vi "Tacking Helper Helper - Waypoint Builder.vi"(4 "Second Arm Length":dbl, 5 "Current Waypoint\nBeing Adjusted":i32, 6 "Starting Arm Length":dbl, 7 "Waypoint\nArray In":T1[](array[typedef]), 9 "Second Angle":dbl, 10 "If true, the starting angle was\nthe last angle used, and will\nbe used first":bool, 11 "Starting Angle":dbl) -> (3 "Waypoint \nArray Out":T1[](array[typedef]))   [LabVIEW 2011]
doc: "This case statement tests whether to use the starting or secondary angle, whatever was used on the last tack. In this way it always returns to center and then continues out on the same path. The correct angle is used to get the x and y coordinates of the corresponding arm, and that is added to the previous waypoint to get the next waypoint in the array."
uses:
  0x2-OCU-Think Comm/0x2 Typedefs/ocuWaypoint.ctl
  0x2-OCU-Think Comm/0x2 Typedefs/waypointTypes.ctl
  2 Typedefs/UTM Location.ctl
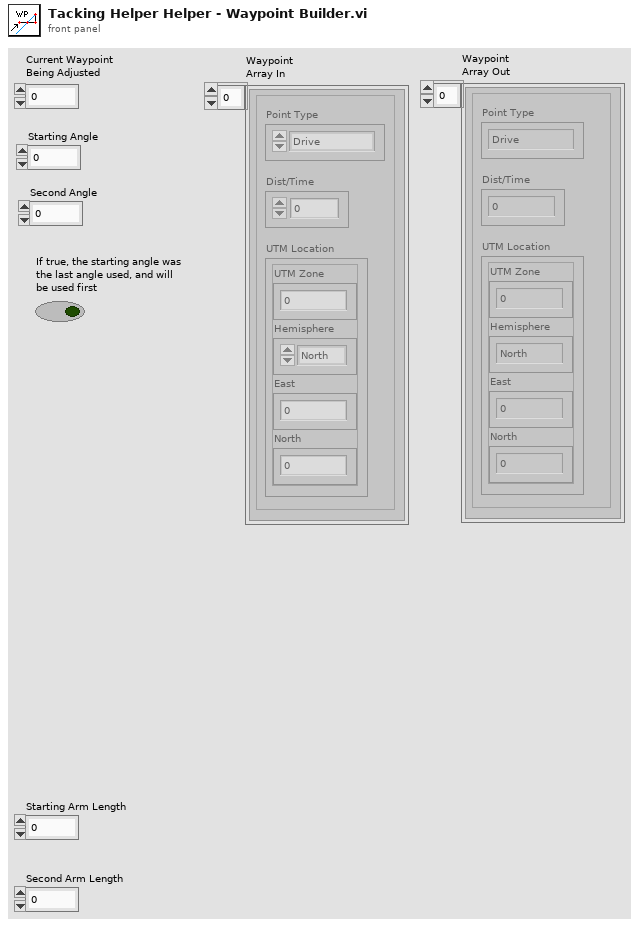
[diagram p1: front panel]
types:
  T1 = typedef "ocuWaypoint.ctl" = cluster{"Point Type":T2, "Dist/Time":dbl, "UTM Location":T3}
  T2 = typedef "waypointTypes.ctl" = enum16{"Drive", "Round Port", "Round Starboard", "Stay"}
  T3 = typedef "UTM Location.ctl" = cluster{"UTM Zone":dbl, "Hemisphere":enum16{"North", "South"}, "East":dbl, "North":dbl}
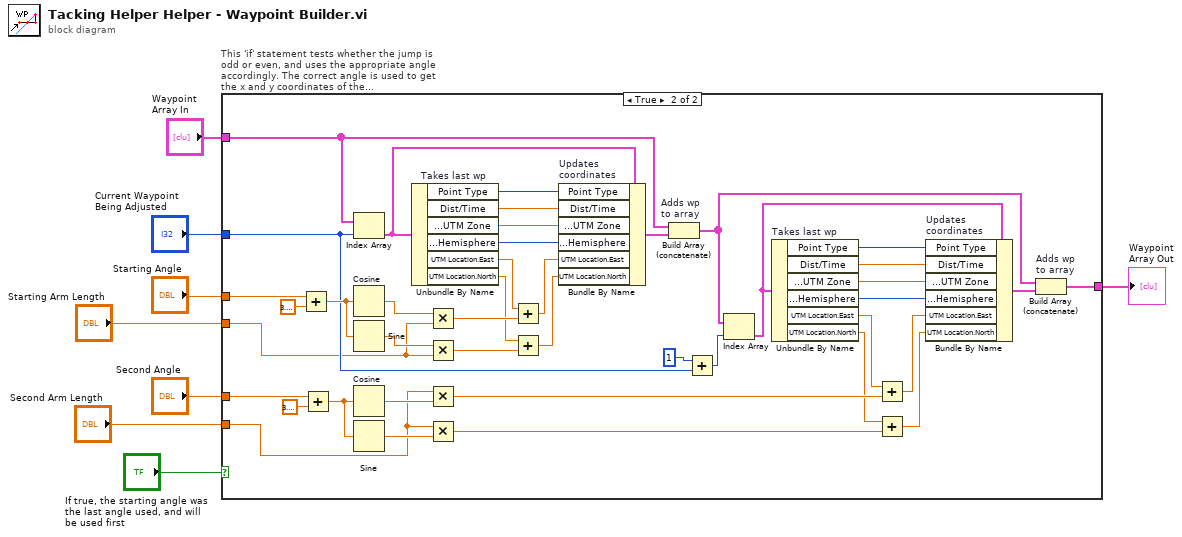
[diagram p0: block diagram]
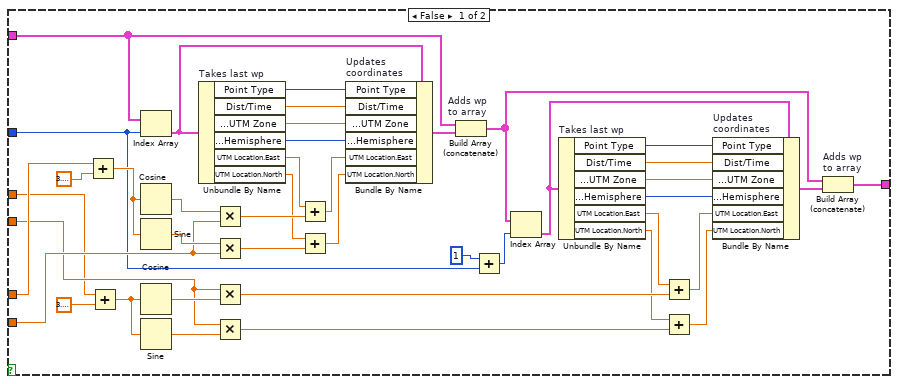
[diagram p2: hidden frame]
diagram:
  n1 = case "This 'if' statement tests whether the jump is odd or even, and uses the appropriate angle accordingly. The correct angle is used to get the x and y coordinates of the\ncorresponding arm, and that is added to the previous waypoint to get the next waypoint in the array." shown="True" "If true, the starting angle was\nthe last angle used, and will\nbe used first" {
    tunnel: "Waypoint\nArray In" -> [w23 w63]
    tunnel: "Current Waypoint\nBeing Adjusted" -> [w11 w55]
    tunnel: "Starting Angle" -> [w9 w87]
    tunnel: "Second Angle" -> [w25 w76]
    tunnel: "Starting Arm Length" -> [w12 w52]
    tunnel: "Second Arm Length" -> [w15 w53]
    tunnel: [w24 w64] -> w8
    frame False {
      n2 = Add(x=w25, y=3.141592653589793) -> (x+y=w43:dbl)
      n3 = Add(x=w9, y=3.141592653589793) -> (x+y=w34:dbl)
      n4 = Index Array(array=w23, index=w11) -> (element=w50:T1)
      n5 = Cosine(x=w43) -> (cos(x)=w14:dbl)
      n6 = Sine(x=w43) -> (sin(x)=w42:dbl)
      n7 = Cosine(x=w34) -> (cos(x)=w13:dbl)
      n8 = Sine(x=w34) -> (sin(x)=w33:dbl)
      n9 = Unbundle By Name "Takes last wp"(w50) -> ("Point Type"=w49:T2, "Dist/Time"=w48:dbl, "UTM Location.UTM Zone"=w47:dbl, "UTM Location.Hemisphere"=w46:enum16{"North", "South"}, "UTM Location.East"=w18:dbl, "UTM Location.North"=w17:dbl)
      n10 = Multiply(x=w14, y=w15) -> (x*y=w19:dbl)
      n11 = Multiply(x=w42, y=w15) -> (x*y=w16:dbl)
      n12 = Multiply(x=w12, y=w13) -> (x*y=w31:dbl)
      n13 = Multiply(x=w12, y=w33) -> (x*y=w32:dbl)
      n14 = Add(x=w18, y=w19) -> (x+y=w44:dbl)
      n15 = Add(x=w17, y=w16) -> (x+y=w41:dbl)
      n16 = Bundle By Name "Updates\ncoordinates"(cluster=w50, "Point Type"=w49, "Dist/Time"=w48, "UTM Location.UTM Zone"=w47, "UTM Location.Hemisphere"=w46, "UTM Location.East"=w44, "UTM Location.North"=w41) -> (w22:T1)
      n17 = Build Array (concatenate) "Adds wp\nto array"(w23, w22) -> (w20:T1[])
      n18 = Add(x=1, y=w11) -> (x+y=w40:i32)
      n19 = Index Array(array=w20, index=w40) -> (element=w26:T1)
      n20 = Unbundle By Name "Takes last wp"(w26) -> ("Point Type"=w39:T2, "Dist/Time"=w38:dbl, "UTM Location.UTM Zone"=w37:dbl, "UTM Location.Hemisphere"=w36:enum16{"North", "South"}, "UTM Location.East"=w30:dbl, "UTM Location.North"=w28:dbl)
      n21 = Add(x=w30, y=w31) -> (x+y=w29:dbl)
      n22 = Add(x=w28, y=w32) -> (x+y=w27:dbl)
      n23 = Bundle By Name "Updates\ncoordinates"(cluster=w26, "Point Type"=w39, "Dist/Time"=w38, "UTM Location.UTM Zone"=w37, "UTM Location.Hemisphere"=w36, "UTM Location.East"=w29, "UTM Location.North"=w27) -> (w21:T1)
      n24 = Build Array (concatenate) "Adds wp\nto array"(w20, w21) -> (w24:T1[])
    }
    frame True {
      n25 = Add(x=w87, y=3.141592653589793) -> (x+y=w84:dbl)
      n26 = Add(x=w76, y=3.141592653589793) -> (x+y=w74:dbl)
      n27 = Index Array(array=w63, index=w55) -> (element=w92:T1)
      n28 = Cosine(x=w84) -> (cos(x)=w51:dbl)
      n29 = Sine(x=w84) -> (sin(x)=w83:dbl)
      n30 = Cosine(x=w74) -> (cos(x)=w73:dbl)
      n31 = Sine(x=w74) -> (sin(x)=w72:dbl)
      n32 = Unbundle By Name "Takes last wp"(w92) -> ("Point Type"=w91:T2, "Dist/Time"=w90:dbl, "UTM Location.UTM Zone"=w89:dbl, "UTM Location.Hemisphere"=w88:enum16{"North", "South"}, "UTM Location.East"=w58:dbl, "UTM Location.North"=w57:dbl)
      n33 = Multiply(x=w51, y=w52) -> (x*y=w59:dbl)
      n34 = Multiply(x=w83, y=w52) -> (x*y=w56:dbl)
      n35 = Multiply(x=w53, y=w73) -> (x*y=w70:dbl)
      n36 = Multiply(x=w53, y=w72) -> (x*y=w71:dbl)
      n37 = Add(x=w58, y=w59) -> (x+y=w85:dbl)
      n38 = Add(x=w57, y=w56) -> (x+y=w82:dbl)
      n39 = Bundle By Name "Updates\ncoordinates"(cluster=w92, "Point Type"=w91, "Dist/Time"=w90, "UTM Location.UTM Zone"=w89, "UTM Location.Hemisphere"=w88, "UTM Location.East"=w85, "UTM Location.North"=w82) -> (w61:T1)
      n40 = Build Array (concatenate) "Adds wp\nto array"(w63, w61) -> (w60:T1[])
      n41 = Add(x=1, y=w55) -> (x+y=w81:i32)
      n42 = Index Array(array=w60, index=w81) -> (element=w65:T1)
      n43 = Unbundle By Name "Takes last wp"(w65) -> ("Point Type"=w80:T2, "Dist/Time"=w79:dbl, "UTM Location.UTM Zone"=w78:dbl, "UTM Location.Hemisphere"=w77:enum16{"North", "South"}, "UTM Location.East"=w69:dbl, "UTM Location.North"=w67:dbl)
      n44 = Add(x=w69, y=w70) -> (x+y=w68:dbl)
      n45 = Add(x=w67, y=w71) -> (x+y=w66:dbl)
      n46 = Bundle By Name "Updates\ncoordinates"(cluster=w65, "Point Type"=w80, "Dist/Time"=w79, "UTM Location.UTM Zone"=w78, "UTM Location.Hemisphere"=w77, "UTM Location.East"=w68, "UTM Location.North"=w66) -> (w62:T1)
      n47 = Build Array (concatenate) "Adds wp\nto array"(w60, w62) -> (w64:T1[])
    }
  }
  "Waypoint \nArray Out" <- w8
